vi "RawFile (configure restart stub.exe).vi"(8 "error in (no error)":errorcluster, 11 "Path to File (empty)":path) -> (0 "error out":errorcluster)   [LabVIEW 2011]
panel:
  in  "FILE":string
  # "Please DO NOT change this control\nname - it gets populated during build."
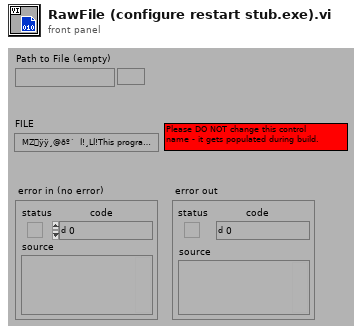
[diagram p1: front panel]
types:
  T1 = enum16{"open", "replace", "create", "open or create", "replace or create", "replace or create with confirmation"}
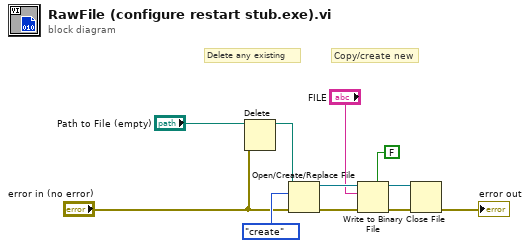
[diagram p0: block diagram]
diagram:
  # "Copy/create new"
  # "Delete any existing"
  n1 = Delete(path (use dialog)="Path to File (empty)", error in="error in (no error)") -> (deleted path=w3:path)  [unwired: 5 out]
  n2 = Open/Create/Replace File(file path (use dialog)=w3, error in="error in (no error)", operation (0:open)=T1."create") -> (refnum out=w8:refnum<file>, error out=w7:errorcluster)  [unwired: 4 out]
  n3 = Write to Binary File(file (use dialog)=w8, data="FILE", error in=w7, 5:FALSE ("prepend array or string size? (T)")) -> (refnum out=w10:refnum<file>, error out=w11:errorcluster)  [unwired: 3 out]
  n4 = Close File(refnum=w10, error in=w11) -> (error out=→"error out":errorcluster)  [unwired: 1 out]
